vi "Requests.vi"(8 "error in (no error)":errorcluster, 9 "write enable":bool=TRUE, 11 "ICPCON ET-7018 in":refnum<class "ICPCON ET-7018.lvclass">) -> (0 "error out":errorcluster, 3 "ICPCON ET-7018 out":refnum<class "ICPCON ET-7018.lvclass">)   [LabVIEW 2021, in "ICPCON ET-7018.lvclass"]
uses:
  ICPCON ET-7018.lvclass
  D:/my_projects/projects/21/Master CR/Master CR.lvclass
  D:/my_projects/projects/21/Master CR/Devices/ET7000/TCP/TCP.lvclass
  Master CR.lvclass/Master CR.ctl
  Modbus_v121c/Modbus Data Unit/Modbus Data Unit.lvclass/Modbus Data Unit.ctl
  Modbus_v121c/Network Protocol/Network Master/Network Master.lvclass/Network Master.ctl
  Modbus_v121c/Master Function Definition/Write Multiple Coils Request.vi
  Modbus_v121c/Master Function Definition/Function data mismatch error.vi
  Modbus_v121c/Master Function Definition/Write Multiple Coils Response.vi
  Modbus_v121c/Network Protocol/Network Master/Read write Master.vi
  Modbus_v121c/Master Function Definition/Read Input Registers Request.vi
  Modbus_v121c/Master Function Definition/Read Input Registers Response.vi
  Modbus_v121c/Master Function Definition/Read Coils Request.vi
  Modbus_v121c/Master Function Definition/Read Coils Response.vi
  Network Protocol/Read Network Protocol.vi
  Modbus_v121c/Modbus Data Unit/Construct PDU.vi
  Modbus_v121c/Utility/Bits to Bytes.vi
  Modbus_v121c/Data Model/Error Generator.vi
  Modbus_v121c/Master Function Definition/Function code mismatch error.vi
  Modbus_v121c/Modbus Data Unit/Deconstruct PDU.vi
  Modbus_v121c/Utility/Bytes to U16s.vi
  Modbus_v121c/Utility/Bytes to Bits.vi
  TCP/TCP.lvclass
  Modbus_v121c/Network Protocol/Network Master/Network Master.lvclass
  Modbus_v121c/Modbus Data Unit/Modbus Data Unit.lvclass
  Modbus_v121c/Data Model/Device Data Model.lvclass
  Modbus_v121c/Transmission Data Unit/Transmission Data Unit.lvclass
  Master CR.lvclass
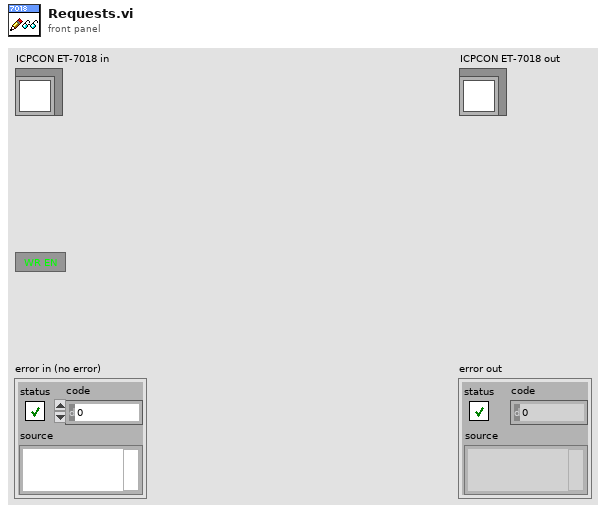
[diagram p1: front panel]
types:
  T1 = typedef "Device Data Model.lvclass/N channel.ctl" = cluster{"N DI channel":i32, "N DO channel":i32, "N AI channel":i32, "N AO channel":i32}
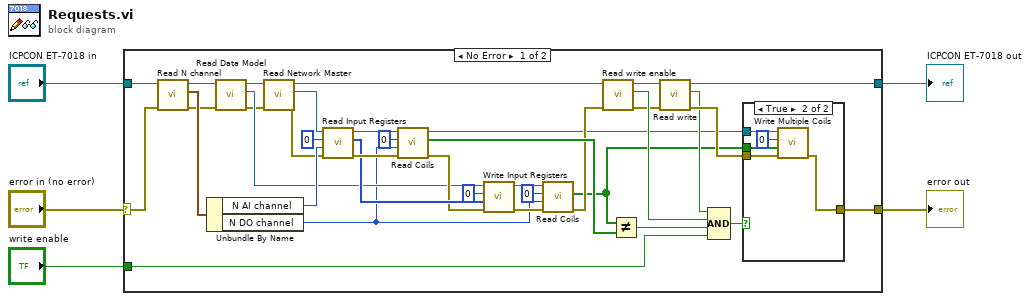
[diagram p0: block diagram]
diagram:
  n1 = case shown="No Error" "error in (no error)" {
    selector: "error in (no error)" -> [w28 w50]
    tunnel: [w41 w50] -> w3
    tunnel: [w12 w49] -> w4
    tunnel: "ICPCON ET-7018 in" -> [w30 w49]
    tunnel: "write enable" -> [w23 _]
    frame No Error {
      n2 = call "Read N channel.vi"("error in (no error)"=w28, "Master CR in"=w30) -> ("error out"=w27:errorcluster, "N channel"=w33:T1, "Master CR out"=w29:refnum<class "ICPCON ET-7018.lvclass">)  [unwired: 7 in]
      n3 = Unbundle By Name(w33) -> ("N AI channel"=w32:i32, "N DO channel"=w16:i32)
      n4 = call "Read Data Model.vi"("error in (no error)"=w27, "Master CR in"=w29) -> ("error out"=w10:errorcluster, "Data Model"=w26:refnum<class "Device Data Model.lvclass">, "Master CR out"=w9:refnum<class "ICPCON ET-7018.lvclass">)  [unwired: 7 in]
      n5 = call "Read Network Master.vi"("error in (no error)"=w10, "TCP in"=w9) -> ("error out"=w8:errorcluster, "Network Master"=w7:refnum<class "Network Master.lvclass">, "TCP out"=w6:refnum<class "ICPCON ET-7018.lvclass">)  [unwired: 7 in]
      n6 = call "Read Input Registers.vi"("error in (no error)"=w8, "number of input registers"=w32, "starting address"=u16 0, "Modbus master in"=w7) -> ("error out"=w38:errorcluster, "register values"=w35:u16[], "Modbus master out"=w39:refnum<class "Network Master.lvclass">)  [unwired: 5 in]
      n7 = call "Read Coils.vi"("error in (no error)"=w38, "number of coils"=w16, "starting address"=u16 0, "Modbus master in"=w39) -> ("error out"=w31:errorcluster, "coil values"=w36:bool[], "Modbus master out"=w11:refnum<class "Network Master.lvclass">)  [unwired: 5 in]
      n8 = call-dynamic "Write Input Registers.vi"("error in (no error)"=w31, "register values"=w35, "starting address"=u16 0, "Device Data Model in"=w26) -> ("error out"=w18:errorcluster, "Device Data Model out"=w17:refnum<class "Device Data Model.lvclass">)  [unwired: 6 in]
      n9 = call-dynamic "Read Coils.vi"("error in"=w18, "number of coils"=w16, "starting address"=u16 0, "device data model in"=w17) -> ("error out"=w14:errorcluster, "data"=w13:bool[])  [unwired: 5 in, 1 out]
      n10 = call "Read write enable.vi"("error in (no error)"=w14, "Master CR in"=w6) -> ("error out"=w21:errorcluster, "write enable"=w24:bool, "Master CR out"=w22:refnum<class "ICPCON ET-7018.lvclass">)  [unwired: 7 in]
      n11 = Not Equal?(x=w13, y=w36) -> (x != y?=w25:bool)
      n12 = call "Read write.vi"("error in (no error)"=w21, "Master CR in"=w22) -> ("error out"=w20:errorcluster, "Write"=w19:bool, "Master CR out"=w12:refnum<class "ICPCON ET-7018.lvclass">)  [unwired: 7 in]
      n13 = Compound Arithmetic op=AND(w19, w24, w25, w23) -> (w42:bool)
      n14 = case shown="True" w42 {
        tunnel: w20 -> [w43 w46]
        tunnel: [w43 w44] -> w41
        tunnel: w13 -> [_ w47]
        tunnel: w11 -> [_ w48]
        frame False {
        }
        frame True {
          n15 = call "Write Multiple Coils.vi"("error in (no error)"=w46, "coil values"=w47, "starting address"=u16 0, "Modbus master in"=w48) -> ("error out"=w44:errorcluster)  [unwired: 6 in, 1 out]
        }
      }
    }
    frame Error {
    }
  }
  "error out" <- w3
  "ICPCON ET-7018 out" <- w4
